vi "Write trust on first use.vi"(8 "error in (no error)":errorcluster, 10 "trust on first use":bool, 11 "Generic Client in":refnum<class "Generic Client.lvclass">) -> (0 "error out":errorcluster, 3 "Generic Client out":refnum<class "Generic Client.lvclass">)   [LabVIEW 2020, in "NI_SSH.lvlib" / "Generic Client.lvclass"]
uses:
  <vilib>/net/SSH/Client/Generic/Generic Client.lvclass
  <vilib>/net/SSH/Client/Generic/Generic Client.lvclass/Generic Client.ctl
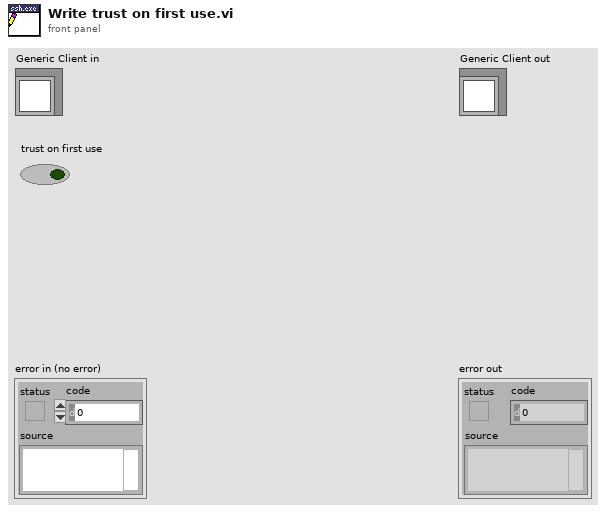
[diagram p1: front panel]
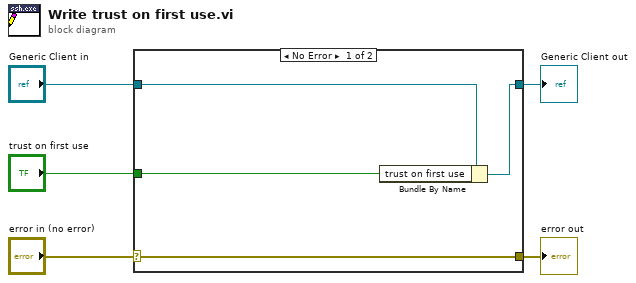
[diagram p0: block diagram]
diagram:
  n1 = case shown="No Error" "error in (no error)" {
    selector: "error in (no error)" -> [w9 w10]
    tunnel: [w9 w10] -> w4
    tunnel: [w7 w11] -> w2
    tunnel: "Generic Client in" -> [w8 w11]
    tunnel: "trust on first use" -> [w6 _]
    frame No Error {
      n2 = Bundle By Name(cluster=w8, "trust on first use"=w6) -> (w7:refnum<class "Generic Client.lvclass">)
    }
    frame Error {
    }
  }
  "error out" <- w4
  "Generic Client out" <- w2
